vi "Multi-channel reverb.vi"(8 "tail length":i32, 9 "fade gain":dbl, 10 "fade delay":i32, 11 "data in":waveform(dbl)[](array[waveform])) -> (3 "data out":waveform(dbl)[](array[waveform]))   [LabVIEW 2023]
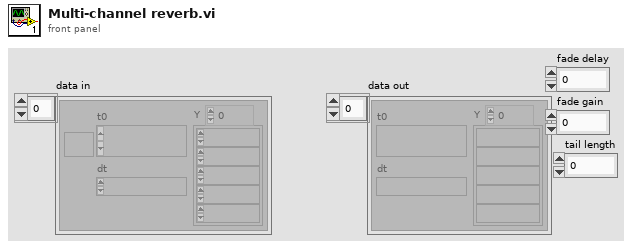
[diagram p1: front panel]
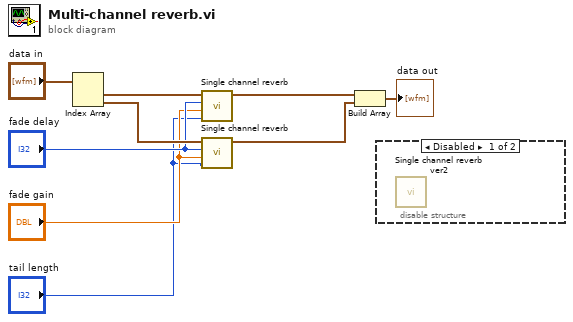
[diagram p0: block diagram]
diagram:
  n1 = Index Array(array="data in") -> (element #1=w6:waveform(dbl), element #2=w5:waveform(dbl))  [unwired: 2 in]
  n2 = call "Single channel reverb.vi"("tail length"="tail length", "fade gain"="fade gain", "fade delay"="fade delay", "data in"=w6) -> ("data out"=w7:waveform(dbl))  [unwired: 7 in]
  n3 = call "Single channel reverb.vi"("tail length"="tail length", "fade gain"="fade gain", "fade delay"="fade delay", "data in"=w5) -> ("data out"=w4:waveform(dbl))  [unwired: 7 in]
  n4 = Build Array(w7, w4) -> (→"data out":waveform(dbl)[])
  n5 = disable-structure shown="Disabled" {
    frame Disabled {
      n6 = call "Single channel reverb ver2.vi"() -> ()  [unwired: 11 in, 1 out]
    }
    frame Enabled {
    }
  }
